vi "TypeDefEnumControls.vi"(7 "Seasons":T3, 10 "Months":T1=enum."December", 11 "Colors":T2=enum."Green") -> ()   [LabVIEW 2012]
uses:
  SeasonsTypeDef.ctl
  ColorsTypeDef.ctl
  MonthsTypeDef.ctl
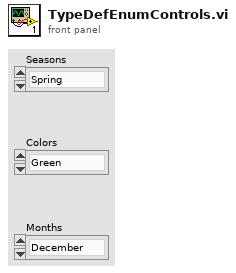
[diagram p1: front panel]
types:
  T1 = typedef "MonthsTypeDef.ctl" = enum32{"<Invalid>", "January", "February", "March", "April", "May", "June", "July", "August", "September", "October", "November", "December"}
  T2 = typedef "ColorsTypeDef.ctl" = enum16{"Red", "Green", "Blue"}
  T3 = typedef "SeasonsTypeDef.ctl" = enum8{"Spring", "Summer", "Fall", "Winter"}
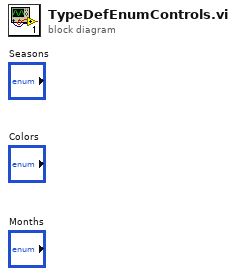
[diagram p0: block diagram]
diagram:
